vi "param (SubVI).vi"(9 "Numeric":bool=TRUE, 11 "Input":string="speed,t") -> (1 "num":i32=2, 2 "parm":dbl[](array[numeric]), 3 "Array":string[](array[string])=["speed", "t"])   [LabVIEW 2014]
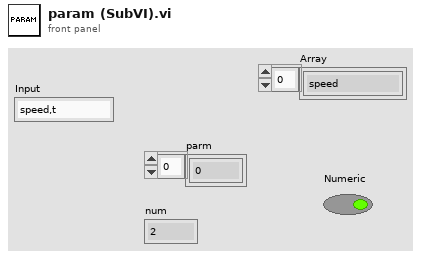
[diagram p1: front panel]
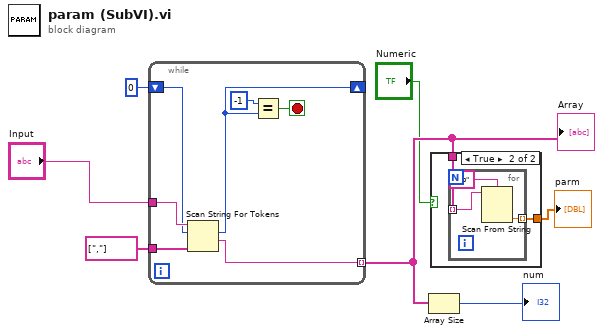
[diagram p0: block diagram]
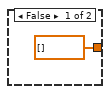
[diagram p2: hidden frame]
diagram:
  n1 = while {
    tunnel: "Input" -> [w14]
    shift-right: [w11] -> _
    shift-left: 0 ("offset of match") -> [w13]
    tunnel: [w12] -> w6 mode=indexing
    tunnel: string[] [","] ("delimiters (\\s,\\t,\\r,\\n)") -> [w9]
    stop <- w8 stop-if-true
    n2 = Scan String For Tokens(6:w9, 8:w13, 9:w14) -> (1:w12:string, 2:w11:i32)  [unwired: 3 in, 2 out]
    n3 = Equal?(x=-1, y=w11) -> (x = y?=w8:bool)
  }
  "Array" <- w6
  n4 = Array Size(array=w6) -> (size(s)=→"num":i32)
  n5 = case shown="True" "Numeric" {
    tunnel: [dbl[] [] w17] -> w7
    tunnel: w6 -> [_ w16]
    frame False {
    }
    frame True {
      n6 = for {
        tunnel: w16 -> [w20] mode=indexing
        tunnel: [w18] -> w17 mode=indexing
        n7 = Scan From String(format string="%p", input string=w20) -> (output 1=w18:dbl)  [unwired: 3 in, 3 out]
      }
    }
  }
  "parm" <- w7
